vi "Control Panel.vi"(8 "error in (no error)":errorcluster, 11 "Level Meter.lvclass":refnum<class "Level Meter.lvclass">) -> (0 "error out":errorcluster, 3 "Magnet.lvclass out":refnum<class "Level Meter.lvclass">)   [LabVIEW 2023, in "Level Meter.lvclass"]
uses:
  Level Meter.lvclass
  Cryogen Levels.ctl
  Utility Classes/InstrPtr/InstrPtr.lvclass
  Level Meter.lvclass/Level Meter.ctl
  Global/Relative Sound Files.vi
  File IO/File IO.lvclass
panel:
  out "Log Counter":dbl
  out "Alarm":bool
  out "*ilm200":T1
  in  "Display last":dbl[unit]=600.0
  out "TX graph":T2(graph)
  in  "Update interval":dbl[unit]=0.1
  in  "Internal UI Refresh":bool
  out "done?":bool
  out "Heliters":dbl caption="LHe Liters" format="%.3f"
  in  "Fast? He":bool
  in  "warningcontN":T3={"alarmliqN"=90.0, "warn?N"=FALSE, "lessthan?N"=FALSE}
  in  "warningcontHe":T4={"alarmliqHe"=85.0, "warn?He"=FALSE, "lessthan?He"=FALSE}
  out "Cryogen Levels":T5 min=-1.0 max=100.0 scale=0.0..100.0
  out "helium":T6 caption="Helium"
  out "nitrogen":cluster{"fillN?":bool, "lowN?":bool} caption="Nitrogen"
  out "shutdown":bool caption="Shut Down"
  out "active":bool
  out "working":bool caption="Working"
  out "ready?":bool
  in  "Refresh":bool
  in  "endprgm":bool
  # "Level Meter Control Panel"
  # "Helium"
  # "Cryogen Levels"
  # "Warning"
  # "Nitrogen"
  # "L"
  # "He Sample Rate"
  # "Slow"
  # "Fast"
  # "Off"
  # "On"
  # "Greater"
  # "Less"
  # "Off"
  # "On"
  # "Greater"
  # "Less"
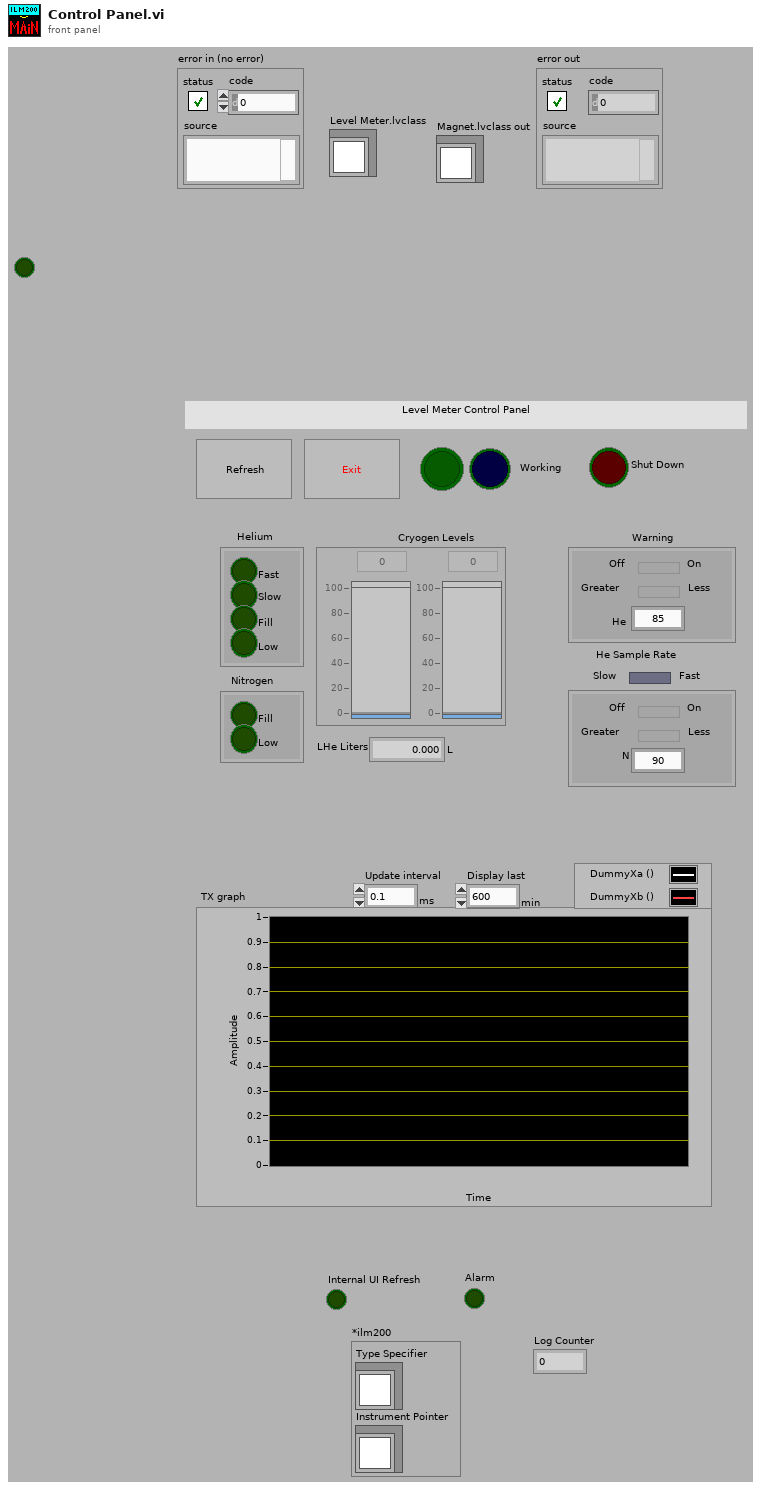
[diagram p1: front panel]
types:
  T1 = cluster{"Type Specifier":refnum<class "Level Meter.lvclass">, "Instrument Pointer":refnum<class "InstrPtr.lvclass">}
  T2 = cluster{"Data Points":cluster{"t":timestamp, "x":dbl}[]}[]
  T3 = cluster{"alarmliqN":dbl, "warn?N":bool, "lessthan?N":bool}
  T4 = cluster{"alarmliqHe":dbl, "warn?He":bool, "lessthan?He":bool}
  T5 = typedef "Level Meter.lvclass/Cryogen Levels.ctl" = dbl[]
  T6 = cluster{"fastHe?":bool, "slowHe?":bool, "fillHe?":bool, "lowHe?":bool}
  T7 = typedef "Readable.lvclass/TX Graph.ctl" = cluster{"Data Points":cluster{"t":timestamp, "x":dbl}[]}[]
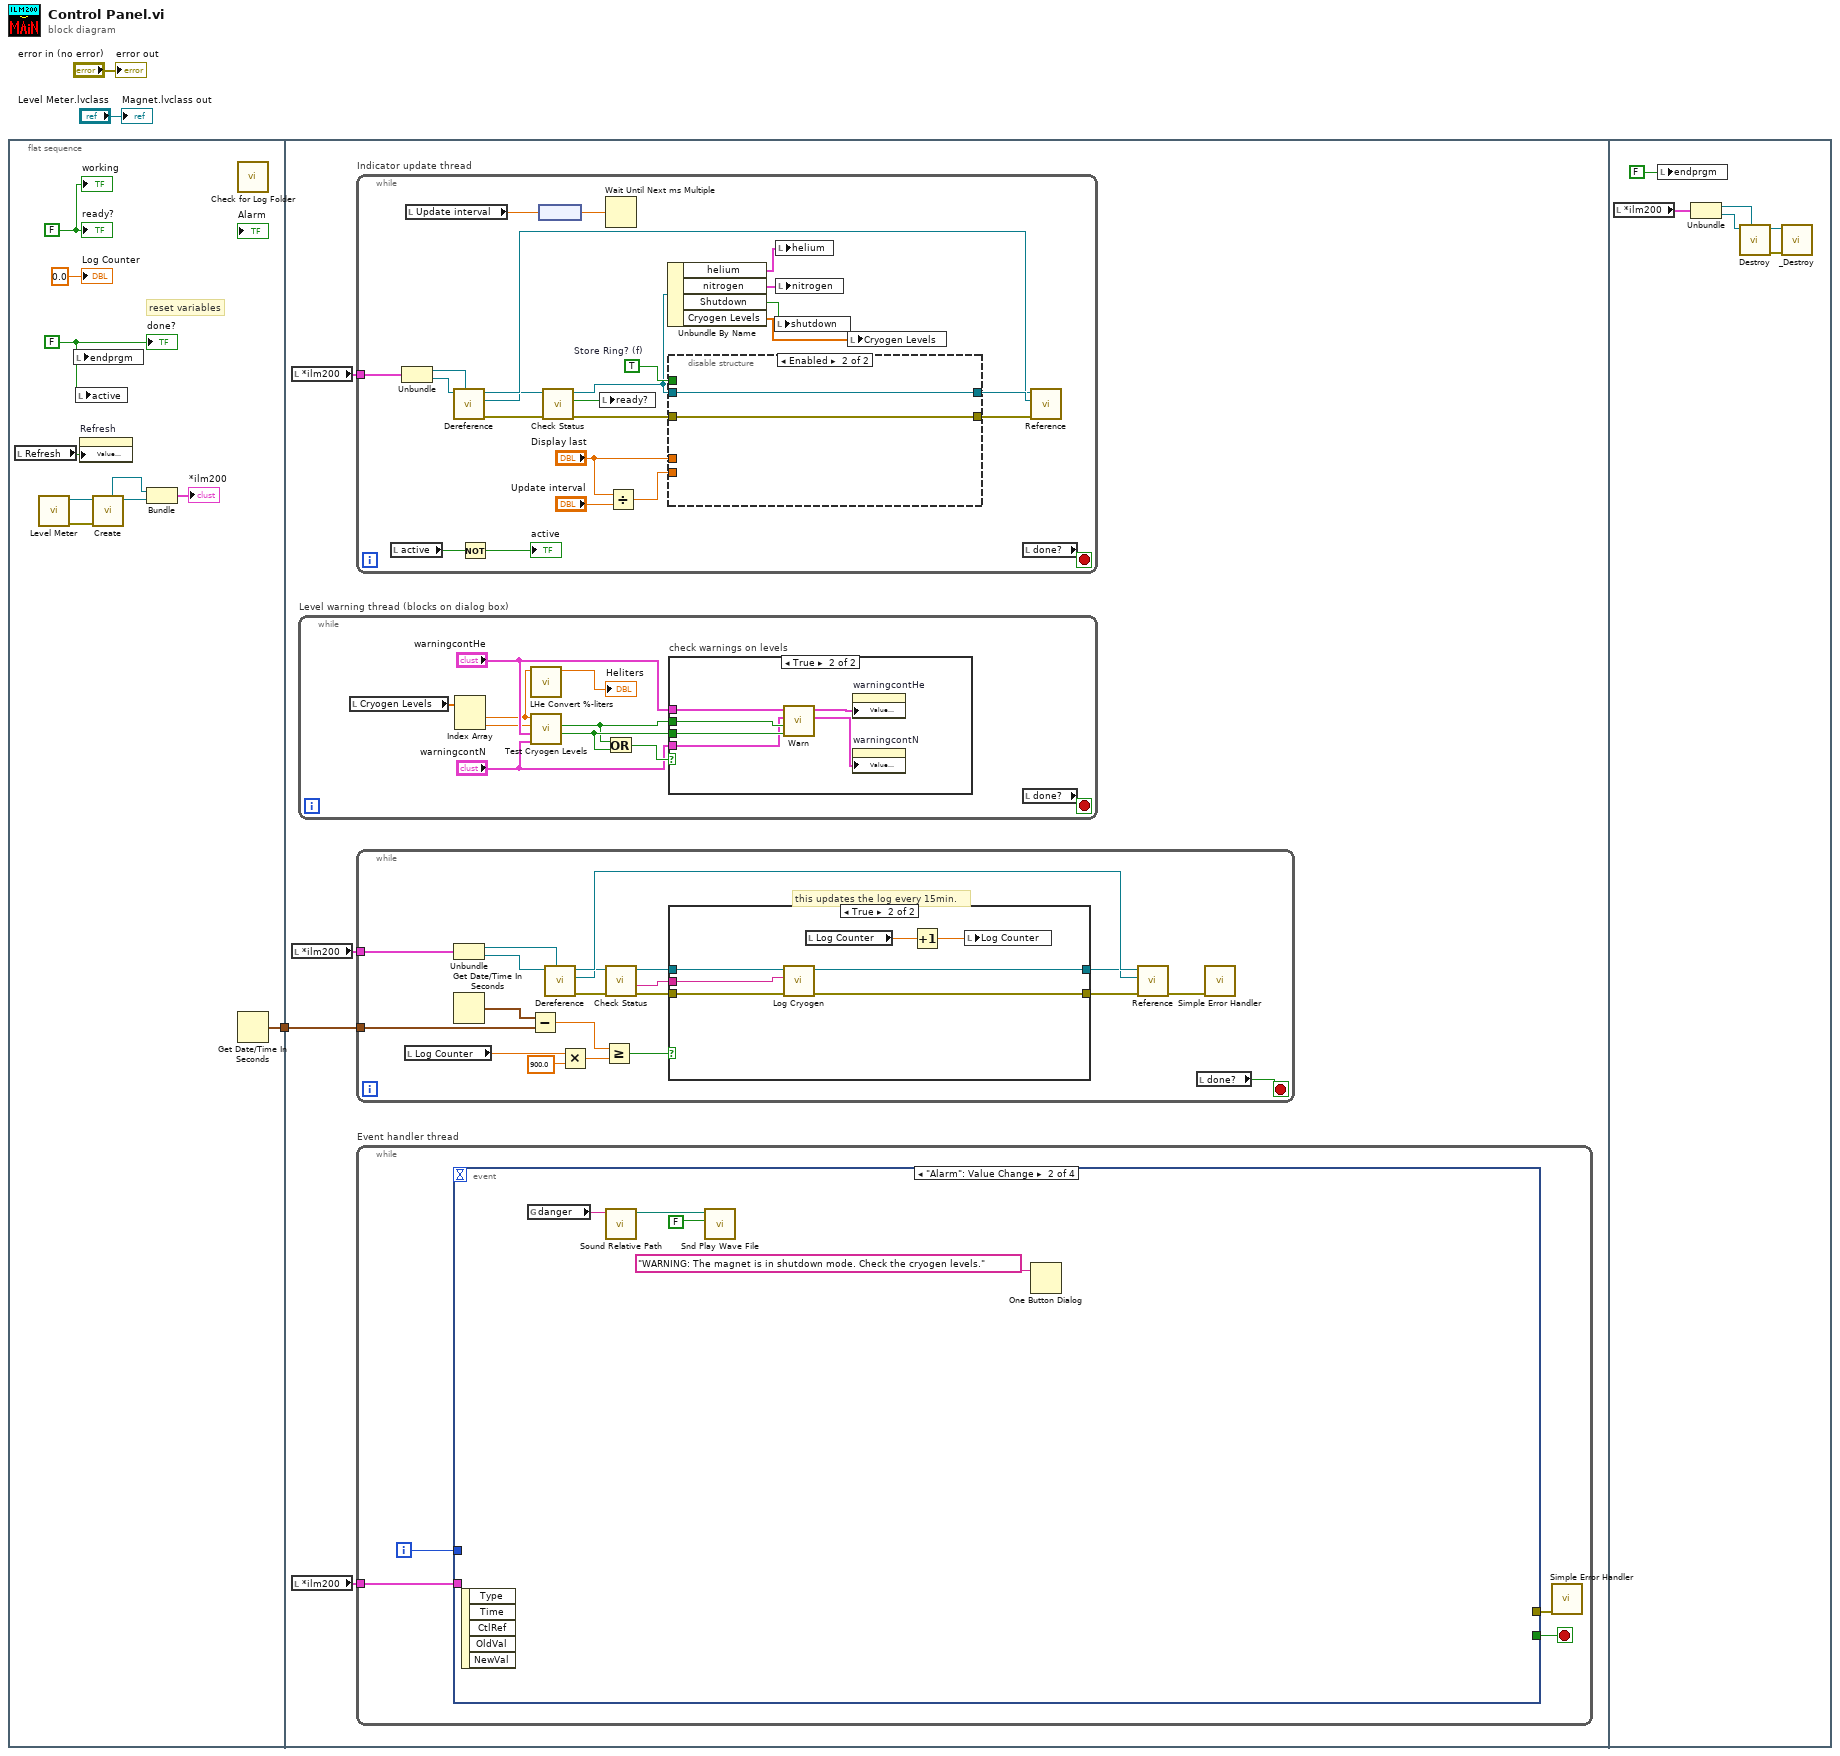
[diagram p0: block diagram]
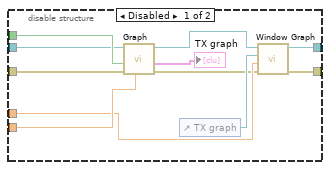
[diagram p4: hidden frame]
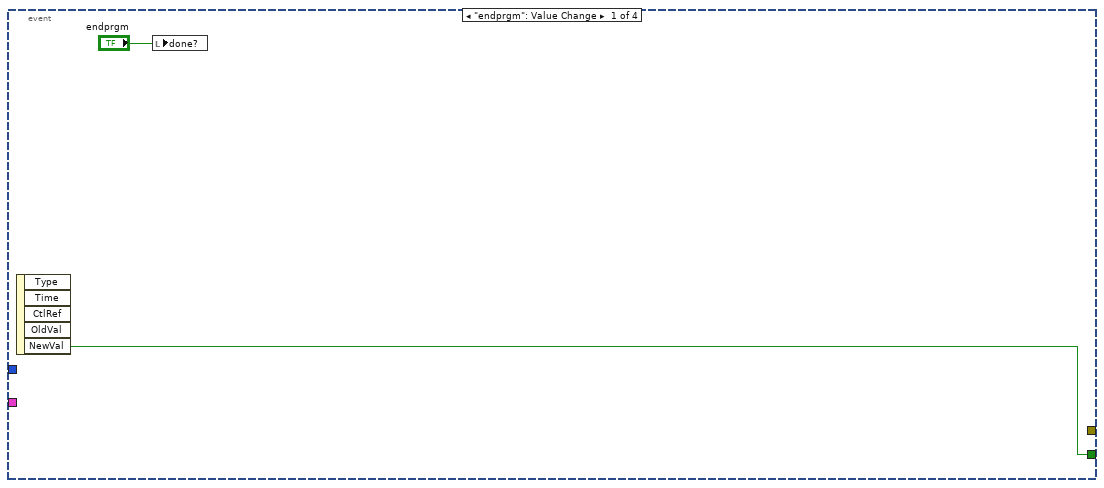
[diagram p5: hidden frame]
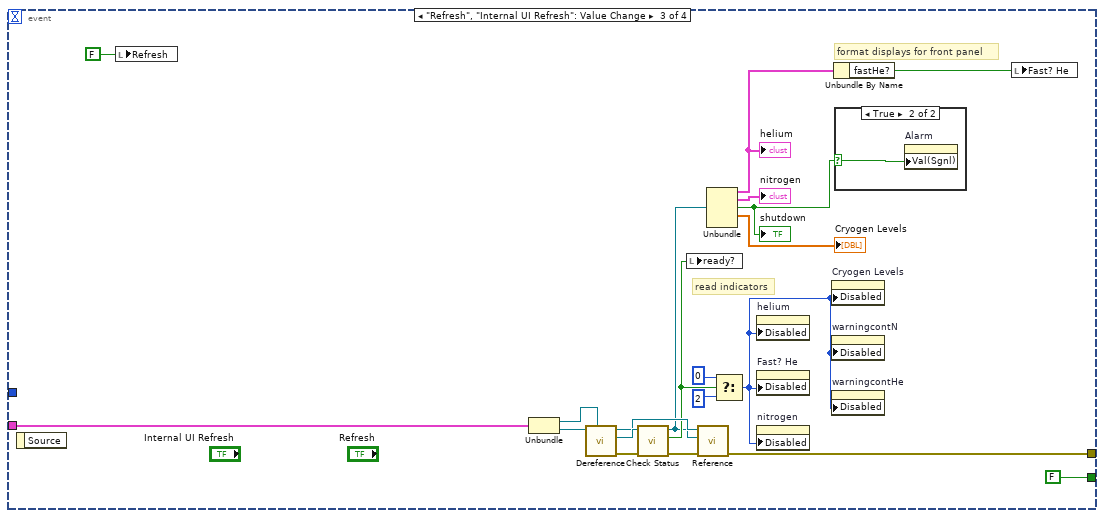
[diagram p6: hidden frame]
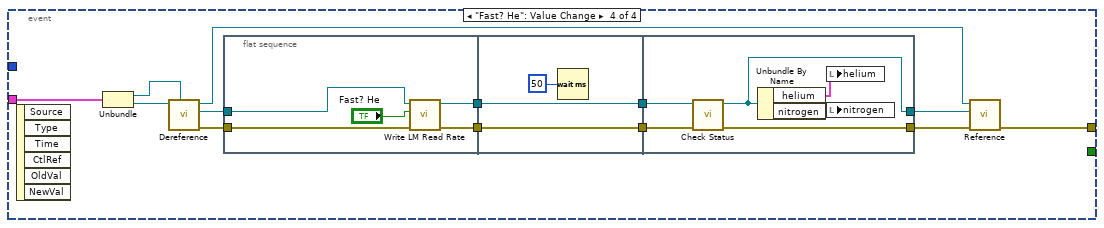
[diagram p8: hidden frame]
diagram:
  n1 = flat-sequence {
    tunnel: [w5] -> w1
    tunnel: w1 -> [w14]
    frame #0 {
      w13 = FALSE
      w11 = FALSE
      # "reset variables"
      n2 = local read "Refresh"() -> (w12:bool)
      n3 = call "Level Meter.vi"() -> ("error out"=w9:errorcluster, "Level Meter out"=w10:refnum<class "Level Meter.lvclass">)  [unwired: 10 in]
      n4 = local write "endprgm"(w11) -> ()
      n5 = local write "active"(w11) -> ()
      n6 = property on="Refresh" class="Bool (strict)"("Value (Signaling)"=w12) -> ()  [unwired: 2 in, 2 out]
      n7 = call "Create.vi"("error in (no error)"=w9, "Instrument in"=w10) -> ("Instrument Pointer"=w8:refnum<class "InstrPtr.lvclass">, "Type Specifier"=w7:refnum<class "Level Meter.lvclass">)  [unwired: 7 in, 1 out]
      n8 = Bundle("Type Specifier"=w7, "Instrument Pointer"=w8) -> (→"*ilm200":T1)  [unwired: 1 in]
      n9 = call "Check for Log Folder.vi"() -> ()  [unwired: 1 out]
      n10 = Get Date/Time In Seconds() -> (seconds since 1Jan1904=w5:timestamp)
      "ready?" <- w13
      "working" <- w13
      "done?" <- w11
      "Log Counter" <- 0.0 ("Log Counter")
    }
    frame #1 {
      n11 = local read "*ilm200"() -> (w17:T1)
      n12 = local read "*ilm200"() -> (w15:T1)
      n13 = local read "*ilm200"() -> (w16:T1)
      n14 = while "Level warning thread (blocks on dialog box)" {
        stop <- w47 stop-if-true
        n15 = local read "Cryogen Levels"() -> (w48:T5)
        n16 = Index Array(array=w48) -> (element #1=w50:dbl, element #2=w49:dbl)  [unwired: 2 in]
        n17 = call "LHe Convert %-liters.vi"("%"=w50) -> ("Lout"=→"Heliters":dbl)  [unwired: 1 in, 9 out]
        n18 = call "Test Cryogen Levels.vi"("warningcontN"="warningcontN", "warningcontHe"="warningcontHe", "LNlevel"=w49, "LHelevel"=w50) -> ("warnN"=w55:bool, "warnHe"=w54:bool)  [unwired: 1 in, 5 out]
        n19 = Or(x=w54, y=w55) -> (x .or. y?=w53:bool)
        n20 = case "check warnings on levels" shown="True" w53 {
          tunnel: w54 -> [_ w62]
          tunnel: w55 -> [_ w61]
          tunnel: "warningcontHe" -> [_ w60]
          tunnel: "warningcontN" -> [_ w59]
          frame False {
          }
          frame True {
            n21 = call "Warn.vi"("NwarnIN"=w61, "HwarnIN"=w62, "warncontN"=w59, "warncontHe"=w60) -> ("warnNOUT"=w58:T3, "warnHeOUT"=w57:T4)  [unwired: 1 in, 5 out]
            n22 = property on="warningcontHe" class="Clust (strict)"("Value (Signaling)"=w57) -> ()  [unwired: 2 in, 2 out]
            n23 = property on="warningcontN" class="Clust (strict)"("Value (Signaling)"=w58) -> ()  [unwired: 2 in, 2 out]
          }
        }
        n24 = local read "done?"() -> (w47:bool)
      }
      n25 = while "Indicator update thread" {
        tunnel: w17 -> [w76]
        stop <- w65 stop-if-true
        w86 = TRUE  # Store Ring? (f)
        n26 = local read "active"() -> (w79:bool)
        n27 = Unbundle(w76) -> ("Type Specifier"=w77:refnum<class "Level Meter.lvclass">, "Instrument Pointer"=w78:refnum<class "InstrPtr.lvclass">)
        n28 = local read "Update interval"() -> (w81:dbl[unit])
        n29 = call "Dereference.vi"("Type Specifier"=w77, "InstrPtr"=w78) -> ("error out"=w67:errorcluster, "Instrument out"=w68:refnum<class "Level Meter.lvclass">, "InstrPtr out"=w74:refnum<class "InstrPtr.lvclass">)  [unwired: 7 in]
        n30 = Not(x=w79) -> (.not. x?=→"active":bool)
        n31 = node(w81) -> (w85:dbl)
        n32 = call-dynamic "Check Status.vi"("error in (no error)"=w67, "Level Meter in"=w68) -> ("error out"=w63:errorcluster, "On?"=w66:bool, "Level Meter out"=w64:refnum<class "Level Meter.lvclass">)  [unwired: 6 in, 1 out]
        n33 = local write "ready?"(w66) -> ()
        n34 = Wait Until Next ms Multiple(millisecond multiple=w85) -> ()  [unwired: 1 out]
        n35 = Divide(x="Display last", y="Update interval") -> (x/y=w83:dbl)
        n36 = Unbundle By Name(w64) -> ("helium"=w69:T6, "nitrogen"=w71:cluster{"fillN?":bool, "lowN?":bool}, "Shutdown"=w70:bool, "Cryogen Levels"=w72:T5)
        n37 = disable-structure shown="Enabled" {
          disable-tunnel: w86 -> [w97 _]
          disable-tunnel: w83 -> [w95 _]
          disable-tunnel: "Display last" -> [w94 _]
          disable-tunnel: w64 -> [w90 w99]
          disable-tunnel: w63 -> [w89 w98]
          disable-tunnel: [w88 w99] -> w75
          disable-tunnel: [w87 w98] -> w73
          frame Disabled {
            n38 = call-dynamic "Graph.vi"("Ring size (points) (1024)"=w95, "error in (no error)"=w89, "Store Ring? (f)"=w97, "Readable in"=w90) -> ("error out"=w91:errorcluster, "Ring Buffers"=→"TX graph":T7, "Readable out"=w92:refnum<class "Level Meter.lvclass">)  [unwired: 3 in, 2 out]
            n39 = control-ref of="TX graph"() -> (w93:refnum<vi>)
            n40 = call-dynamic "Window Graph.vi"("error in (no error)"=w91, "Window"=w94, "Graph ref"=w93, "Readable in"=w92) -> ("error out"=w87:errorcluster, "Readable out"=w88:refnum<class "Level Meter.lvclass">)  [unwired: 6 in]
          }
          frame Enabled {
          }
        }
        n41 = local write "shutdown"(w70) -> ()
        n42 = local write "helium"(w69) -> ()
        n43 = local write "nitrogen"(w71) -> ()
        n44 = local write "Cryogen Levels"(w72) -> ()
        n45 = local read "done?"() -> (w65:bool)
        n46 = call "Reference.vi"("error in (no error)"=w73, "Instrument"=w75, "InstrPtr in"=w74) -> ()  [unwired: 8 in, 1 out]
      }
      n47 = while {
        tunnel: w15 -> [w31]
        tunnel: w14 -> [w22]
        stop <- w37 stop-if-true
        # "this updates the log every 15min."
        n48 = local read "Log Counter"() -> (w20:dbl)
        n49 = Unbundle(w31) -> ("Type Specifier"=w30:refnum<class "Level Meter.lvclass">, "Instrument Pointer"=w29:refnum<class "InstrPtr.lvclass">)
        n50 = Get Date/Time In Seconds() -> (seconds since 1Jan1904=w23:timestamp)
        n51 = Subtract(x=w23, y=w22) -> (x-y=w19:dbl)
        n52 = call "Dereference.vi"("Type Specifier"=w30, "InstrPtr"=w29) -> ("error out"=w36:errorcluster, "Instrument out"=w27:refnum<class "Level Meter.lvclass">, "InstrPtr out"=w28:refnum<class "InstrPtr.lvclass">)  [unwired: 7 in]
        n53 = Multiply(x=w20, y=900.0 ("millisecond multiple")) -> (x*y=w18:dbl)
        n54 = Greater Or Equal?(x=w19, y=w18) -> (x >= y?=w24:bool)
        n55 = call-dynamic "Check Status.vi"("error in (no error)"=w36, "Level Meter in"=w27) -> ("error out"=w35:errorcluster, "Status"=w34:string, "Level Meter out"=w33:refnum<class "Level Meter.lvclass">)  [unwired: 6 in, 1 out]
        n56 = case shown="True" w24 {
          tunnel: w35 -> [w38 w46]
          tunnel: w34 -> [_ w45]
          tunnel: w33 -> [w39 w44]
          tunnel: [w38 w43] -> w32
          tunnel: [w39 w42] -> w26
          frame False {
          }
          frame True {
            n57 = call-dynamic "Log Cryogen.vi"("error in (no error)"=w46, "Status string"=w45, "Level Meter in"=w44) -> ("error out"=w43:errorcluster, "Level Meter out"=w42:refnum<class "Level Meter.lvclass">)  [unwired: 7 in]
            n58 = local read "Log Counter"() -> (w41:dbl)
            n59 = Increment(x=w41) -> (x+1=w40:dbl)
            n60 = local write "Log Counter"(w40) -> ()
          }
        }
        n61 = call "Reference.vi"("error in (no error)"=w32, "Instrument"=w26, "InstrPtr in"=w28) -> ("error out"=w25:errorcluster)  [unwired: 8 in]
        n62 = local read "done?"() -> (w37:bool)
        n63 = call <vilib>:"Simple Error Handler.vi"("error in (no error)"=w25) -> ()  [unwired: 4 in, 5 out]
      }
      n64 = while "Event handler thread" {
        tunnel: w16 -> [w101]
        i -> [w102]
        stop <- w103 stop-if-true
        n65 = event shown="[1] \"Alarm\": Value Change" {
          selector: _ -> [_ _ _ _]
          dyn-events: _ -> [_ _ _ _]
          timeout: _ -> [_ _ _ _]
          tunnel: [w105 _ FALSE _] -> w103
          tunnel: w102 -> [_ _ _ _]
          tunnel: w101 -> [_ _ w125 w141]
          tunnel: [_ _ w122 w131] -> w100
          event "endprgm": Value Change {
            n66 = event-data() -> ("NewVal"=w105:bool)  [unwired: 5 out]
            n67 = local write "done?"("endprgm") -> ()
          }
          event "Alarm": Value Change {
            n68 = event-data() -> ()  [unwired: 6 out]
            n69 = global read "Relative Sound Files.vi" "danger"() -> (w108:string)
            n70 = call "Sound Relative Path.vi"("Sound"=w108) -> ("Relative Path"=w107:path)  [unwired: 10 in]
            n71 = call <vilib>:"Snd Play Wave File.vi"("wait until finish (T)"=FALSE, "wave file path"=w107) -> ()  [unwired: 1 in, 9 out]
            n72 = One Button Dialog(message="WARNING: The magnet is in shutdown mode. Check the cryogen levels.") -> ()  [unwired: 1 in, 1 out]
          }
          event "Refresh", "Internal UI Refresh": Value Change {
            # "format displays for front panel"
            # "read indicators"
            n73 = event-data() -> ()  [unwired: 2 out]
            n74 = local write "Refresh"(FALSE) -> ()
            n75 = Unbundle(w125) -> ("Type Specifier"=w127:refnum<class "Level Meter.lvclass">, "Instrument Pointer"=w126:refnum<class "InstrPtr.lvclass">)
            n76 = call "Dereference.vi"("Type Specifier"=w127, "InstrPtr"=w126) -> ("error out"=w121:errorcluster, "Instrument out"=w124:refnum<class "Level Meter.lvclass">, "InstrPtr out"=w123:refnum<class "InstrPtr.lvclass">)  [unwired: 7 in]
            n77 = call-dynamic "Check Status.vi"("error in (no error)"=w121, "Level Meter in"=w124) -> ("error out"=w112:errorcluster, "On?"=w117:bool, "Level Meter out"=w111:refnum<class "Level Meter.lvclass">)  [unwired: 6 in, 1 out]
            n78 = local write "ready?"(w117) -> ()
            n79 = call "Reference.vi"("error in (no error)"=w112, "Instrument"=w111, "InstrPtr in"=w123) -> ("error out"=w122:errorcluster)  [unwired: 8 in]
            n80 = Unbundle(w111) -> (w114:T6, →"nitrogen":cluster{"fillN?":bool, "lowN?":bool}, w110:bool, →"Cryogen Levels":T5)  [unwired: 1 out]
            "helium" <- w114
            "shutdown" <- w110
            n81 = Select(t=0, s=w117, f=2) -> (s? t:f=w118:i32)
            n82 = property on="helium" class="Clust (strict)"("Disabled"=w118) -> ()  [unwired: 2 in, 2 out]
            n83 = property on="Fast? He" class="Bool (strict)"("Disabled"=w118) -> ()  [unwired: 2 in, 2 out]
            n84 = property on="nitrogen" class="Clust (strict)"("Disabled"=w118) -> ()  [unwired: 2 in, 2 out]
            n85 = property on="Cryogen Levels" class="Arr (strict)"("Disabled"=w118) -> ()  [unwired: 2 in, 2 out]
            n86 = property on="warningcontN" class="Clust (strict)"("Disabled"=w118) -> ()  [unwired: 2 in, 2 out]
            n87 = property on="warningcontHe" class="Clust (strict)"("Disabled"=w118) -> ()  [unwired: 2 in, 2 out]
            n88 = Unbundle By Name(w114) -> ("fastHe?"=w113:bool)
            n89 = case shown="True" w110 {
              selector: w110 -> [_ w130]
              frame False {
              }
              frame True {
                n90 = property on="Alarm" class="Bool (strict)"("Val(Sgnl)"=w130) -> ()  [unwired: 2 in, 2 out]
              }
            }
            n91 = local write "Fast? He"(w113) -> ()
          }
          event "Fast? He": Value Change {
            n92 = event-data() -> ()  [unwired: 7 out]
            n93 = Unbundle(w141) -> ("Type Specifier"=w143:refnum<class "Level Meter.lvclass">, "Instrument Pointer"=w142:refnum<class "InstrPtr.lvclass">)
            n94 = call "Dereference.vi"("Type Specifier"=w143, "InstrPtr"=w142) -> ("error out"=w135:errorcluster, "Instrument out"=w136:refnum<class "Level Meter.lvclass">, "InstrPtr out"=w140:refnum<class "InstrPtr.lvclass">)  [unwired: 7 in]
            n95 = flat-sequence {
              tunnel: [w147] -> w138
              tunnel: w136 -> [w146]
              tunnel: w135 -> [w145]
              tunnel: [w144] -> w133
              tunnel: w138 -> [w150]
              tunnel: [w150] -> w137
              tunnel: [w149] -> w134
              tunnel: w133 -> [w149]
              tunnel: [w155] -> w139
              tunnel: w137 -> [w154]
              tunnel: w134 -> [w153]
              tunnel: [w152] -> w132
              frame #0 {
                n96 = call-dynamic "Write LM Read Rate.vi"("error in (no error)"=w145, "Fast?"="Fast? He", "Level Meter in"=w146) -> ("error out"=w144:errorcluster, "Level Meter out"=w147:refnum<class "Level Meter.lvclass">)  [unwired: 7 in]
              }
              frame #1 {
                n97 = Wait (ms)(milliseconds to wait=50) -> ()  [unwired: 1 out]
              }
              frame #2 {
                n98 = call-dynamic "Check Status.vi"("error in (no error)"=w153, "Level Meter in"=w154) -> ("error out"=w152:errorcluster, "Level Meter out"=w155:refnum<class "Level Meter.lvclass">)  [unwired: 6 in, 2 out]
                n99 = Unbundle By Name(w155) -> ("helium"=w157:T6, "nitrogen"=w156:cluster{"fillN?":bool, "lowN?":bool})
                n100 = local write "helium"(w157) -> ()
                n101 = local write "nitrogen"(w156) -> ()
              }
            }
            n102 = call "Reference.vi"("error in (no error)"=w132, "Instrument"=w139, "InstrPtr in"=w140) -> ("error out"=w131:errorcluster)  [unwired: 8 in]
          }
        }
        n103 = call <vilib>:"Simple Error Handler.vi"("error in (no error)"=w100) -> ()  [unwired: 4 in, 5 out]
      }
    }
    frame #2 {
      n104 = local read "*ilm200"() -> (w160:T1)
      n105 = local write "endprgm"(FALSE) -> ()
      n106 = Unbundle(w160) -> ("Type Specifier"=w159:refnum<class "Level Meter.lvclass">, "Instrument Pointer"=w158:refnum<class "InstrPtr.lvclass">)
      n107 = call "Destroy.vi"("Type Specifier"=w159, "InstrPtr in"=w158) -> ("error out"=w162:errorcluster, "final Instrument"=w161:refnum<class "Level Meter.lvclass">)  [unwired: 8 in]
      n108 = call-dynamic "_Destroy.vi"("error in (no error)"=w162, "Instrument in"=w161) -> ()  [unwired: 9 in, 1 out]
    }
  }
  "Magnet.lvclass out" <- "Level Meter.lvclass"
  "error out" <- "error in (no error)"
